vi "AGCxxx Initialize.vi"(0 "AGCxxx VISA Cluster":T1={"VISA resource name"="", "VISA Timeout Value (1000 ms)"=1000, "Lock Timeout (1000 ms)"=1000, "MAX Channel (6)"=6}, 5 "ID Query (T: Check)":bool=TRUE, 7 "Reset (T: Reset)":bool=TRUE, 9 "access mode":u32, 11 "error in (no error)":errorcluster, 12 "Open timeout (1000ms)":u32=1000) -> (4 "dup AGCxxx VISA Cluster":T1={"VISA resource name"="", "VISA Timeout Value (1000 ms)"=1000, "Lock Timeout (1000 ms)"=1000, "MAX Channel (6)"=6}, 15 "error out":errorcluster)   [LabVIEW 2014, in "AGCxxx - Driver.lvlib"]
doc: "This VI passes the addressing information in the instrument decriptor to the Instr Open VI and returns the instrument ID. You can optionally reset the instrument by setting the front panel reset control. You must run this VI before using any of the instrument driver VIs for this instrument.\n! THE AGC NEEDS 12 SECONDS TO RESET !\n\nCopyright (C) \nGesellschaft f. Schwerionenforschung, GSI\nPlanckstr. 1\n64291 Darmstadt\nGermany\n\nContact: http://www-wnt.gsi.de/labview\n H.Brand@gsi.de\n\nThis program is free software; you can redistribute it and/or\nmodify it under the terms of the GNU General Public License\nas published by the Free Software Foundation; either version 2\nof the License, or (at your option) any later version.\n\nThis program is distributed in the hope that it will be useful,\nbut WITHOUT ANY WARRANTY; without even the implied warranty of\nMERCHANTABILITY or FITNESS FOR A PARTICULAR PURPOSE. See the\nGNU General Public License for more details (http://www.gnu.org)."
uses:
  AGCxxx - Driver.lvlib
  AGCxxx VISA Control.ctl
panel:
  in  "Case Constant\n(See Context Help)":bool
  # "Check\nDon't Check"
  # "Reset\nDon't Reset"
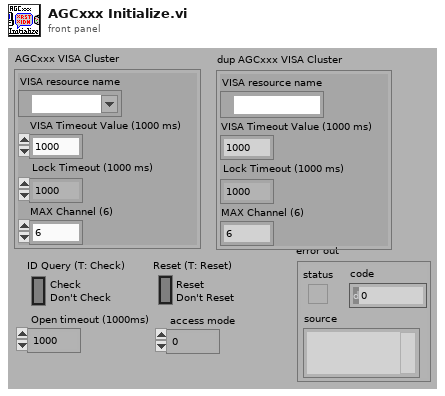
[diagram p1: front panel]
types:
  T1 = typedef "AGCxxx - Driver.lvlib/AGCxxx VISA Control.ctl" = cluster{"VISA resource name":refnum<visa-resource-name>, "VISA Timeout Value (1000 ms)":u32, "Lock Timeout (1000 ms)":u32, "MAX Channel (6)":i32}
  T2 = cluster{"Status":bool, "Code":i32, "Source (VI Name)":string}
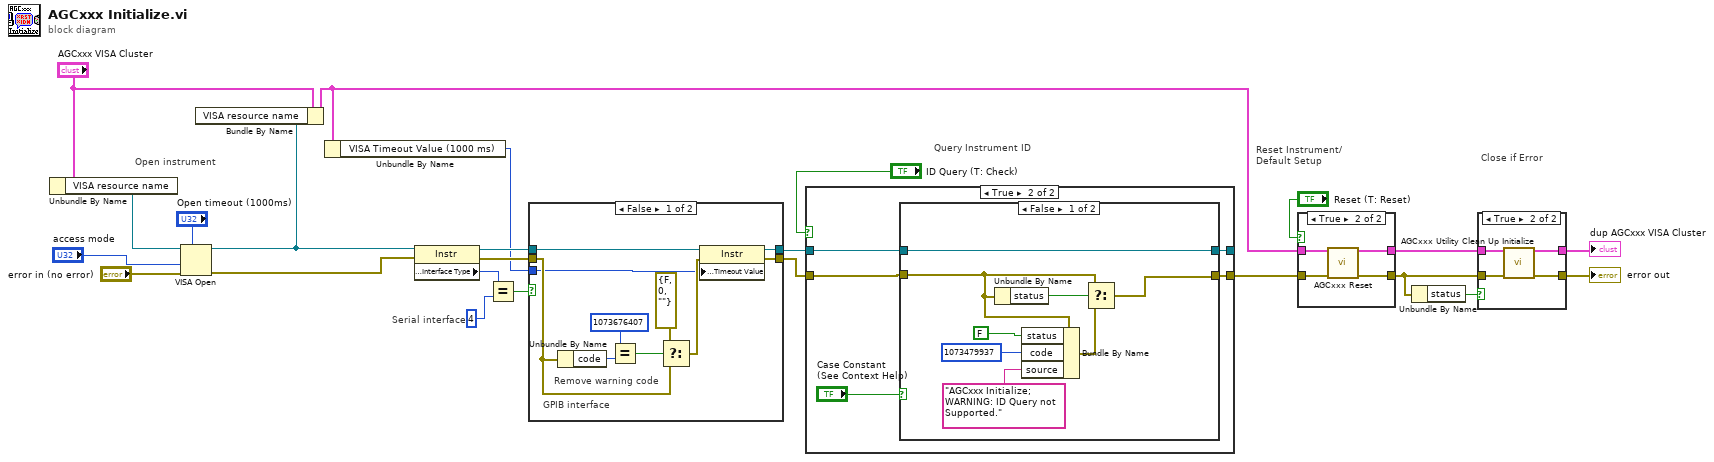
[diagram p0: block diagram]
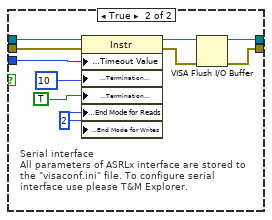
[diagram p2: hidden frame]
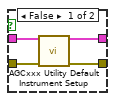
[diagram p4: hidden frame]
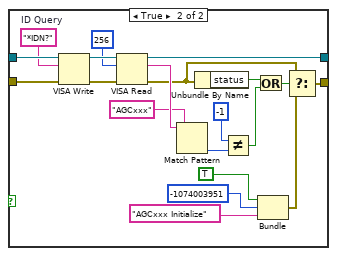
[diagram p6: hidden frame]
diagram:
  # "Serial interface"
  # "Close if Error"
  # "Query Instrument ID"
  # "Reset Instrument/\nDefault Setup"
  # "Open instrument"
  n1 = Unbundle By Name("AGCxxx VISA Cluster") -> ("VISA resource name"=w7:refnum<visa-resource-name>)
  n2 = VISA Open(timeout (0)="Open timeout (1000ms)", access mode="access mode", error in (no error)="error in (no error)", VISA resource name=w7) -> (VISA resource name=w3:refnum<visa-resource-name>, error out=w6:errorcluster)  [unwired: 1 in]
  n3 = Bundle By Name(cluster="AGCxxx VISA Cluster", "VISA resource name"=w3) -> (w2:T1)
  n4 = Unbundle By Name(w2) -> ("VISA Timeout Value (1000 ms)"=w5:u32)
  n5 = property class="Instr"(reference=w3, error in=w6) -> (reference out=w14:refnum<visa-resource-name>, error out=w15:errorcluster, "Interface Information:Interface Type"=w17:u16)
  n6 = Equal?(x=w17, y=u16 4) -> (x = y?=w16:bool)
  n7 = case shown="False" w16 {
    tunnel: w15 -> [w27 w43]
    tunnel: w14 -> [w34 w44]
    tunnel: [w33 w36] -> w12
    tunnel: [w32 w38] -> w11
    tunnel: w5 -> [w25 w35]
    frame False {
      # "Remove warning code"
      # "GPIB interface"
      n8 = Unbundle By Name(w27) -> ("code"=w28:i32)
      n9 = Equal?(x=1073676407, y=w28) -> (x = y?=w30:bool)
      n10 = Select(t=errorcluster {"status"=FALSE, "code"=0, "source"=""} ("error out"), s=w30, f=w27) -> (s? t:f=w26:errorcluster)
      n11 = property class="Instr"(reference=w34, error in=w26, "General Settings:Timeout Value"=w25) -> (reference out=w32:refnum<visa-resource-name>, error out=w33:errorcluster)
    }
    frame True {
      w40 = u16 2 ("ASRL End In")
      # "Serial interface\nAll parameters of ASRLx interface are stored to the \"visaconf.ini\" file. To configure serial interface use please T&M Explorer."
      n12 = property class="Instr"(reference=w44, error in=w43, "General Settings:Timeout Value"=w35, "Message Based Settings:Termination Character"=u8 10 ("TermChar"), "Message Based Settings:Termination Character Enable"=TRUE ("TermChar En"), "Serial Settings:End Mode for Reads"=w40, "Serial Settings:End Mode for Writes"=w40) -> (reference out=w39:refnum<visa-resource-name>, error out=w37:errorcluster)
      n13 = VISA Flush I/O Buffer(VISA resource name=w39, error in (no error)=w37) -> (VISA resource name out=w38:refnum<visa-resource-name>, error out=w36:errorcluster)  [unwired: 1 in]
    }
  }
  n14 = case shown="True" "ID Query (T: Check)" {
    tunnel: [w45 w51] -> w24
    tunnel: [w46 w48] -> _
    tunnel: w11 -> [w46 w49]
    tunnel: w12 -> [w45 w50]
    frame False {
    }
    frame True {
      n15 = case shown="False" "Case Constant\n(See Context Help)" {
        tunnel: [w53 w76] -> w48
        tunnel: w49 -> [w53 w74]
        tunnel: w50 -> [w54 w71]
        tunnel: [w52 w62] -> w51
        frame False {
          n16 = Unbundle By Name(w54) -> ("status"=w56:bool)
          n17 = Bundle By Name(cluster=w54, "status"=FALSE, "code"=1073479937, "source"="AGCxxx Initialize;  WARNING: ID Query not Supported.") -> (w55:errorcluster)
          n18 = Select(t=w54, s=w56, f=w55) -> (s? t:f=w52:errorcluster)
        }
        frame True {
          w64 = "*IDN?"  # ID Query
          n19 = VISA Write(VISA resource name=w74, write buffer=w64, error in (no error)=w71) -> (VISA resource name out=w75:refnum<visa-resource-name>, error out=w72:errorcluster)  [unwired: 1 out]
          n20 = VISA Read(VISA resource name=w75, byte count=u32 256, error in (no error)=w72) -> (VISA resource name out=w76:refnum<visa-resource-name>, read buffer=w77:string, error out=w73:errorcluster)  [unwired: 1 out]
          n21 = Match Pattern(string=w77, regular expression="AGCxxx") -> (offset past match=w66:i32)  [unwired: 1 in, 3 out]
          n22 = Unbundle By Name(w73) -> ("status"=w69:bool)
          n23 = Not Equal?(x=-1, y=w66) -> (x != y?=w78:bool)
          n24 = Or(x=w69, y=w78) -> (x .or. y?=w70:bool)
          n25 = Bundle("Status"=TRUE, "Code"=-1074003951, "Source (VI Name)"="AGCxxx Initialize") -> (w63:T2)  [unwired: 1 in]
          n26 = Select(t=w73, s=w70, f=w63) -> (s? t:f=w62:T2)
        }
      }
    }
  }
  n27 = case shown="True" "Reset (T: Reset)" {
    tunnel: w24 -> [w82 w84]
    tunnel: [w81 w87] -> w20
    tunnel: w2 -> [w83 w85]
    tunnel: [w80 w86] -> w19
    frame False {
      n28 = call "AGCxxx Utility Default Instrument Setup.vi"("AGCxxx VISA Cluster"=w83, "error in (no error)"=w82) -> ("dup AGCxxx VISA Cluster"=w80:T1, "error out"=w81:errorcluster)  [unwired: 12 in]
    }
    frame True {
      n29 = call "AGCxxx Reset.vi"("AGCxxx VISA Cluster"=w85, "error in (no error)"=w84) -> ("dup AGCxxx VISA Cluster"=w86:T1, "error out"=w87:errorcluster)  [unwired: 12 in]
    }
  }
  n30 = Unbundle By Name(w20) -> ("status"=w21:bool)
  n31 = case shown="True" w21 {
    tunnel: w19 -> [w89 w93]
    tunnel: w20 -> [w88 w92]
    tunnel: [w89 w91] -> w1
    tunnel: [w88 w90] -> w18
    frame False {
    }
    frame True {
      n32 = call "AGCxxx Utility Clean Up Initialize.vi"("AGCxxx VISA Cluster"=w93, "error in (no error)"=w92) -> ("dup AGCxxx VISA Cluster"=w91:T1, "error out"=w90:errorcluster)  [unwired: 12 in]
    }
  }
  "error out" <- w18
  "dup AGCxxx VISA Cluster" <- w1
